vi "test_FirstSessionCloseErrors_CallCloseSessions_CloseCalledForAllSessions.vi"(8 "error in":errorcluster) -> (0 "error out":errorcluster, 2 "result":string, 3 "pass":bool)   [LabVIEW 2020, in "MeasurementServerTests.lvlib"]
uses:
  MeasurementServerTests.lvlib
  Runtime/Clients/Session Management V1/Session Reservation/Session Reservation.lvclass
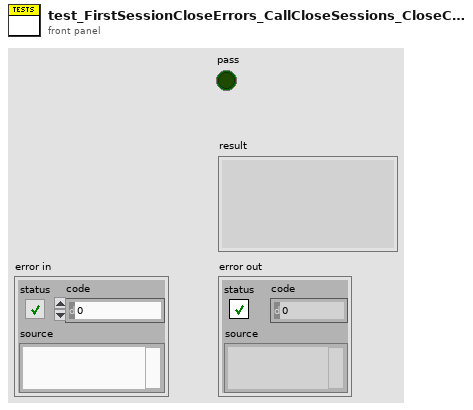
[diagram p1: front panel]
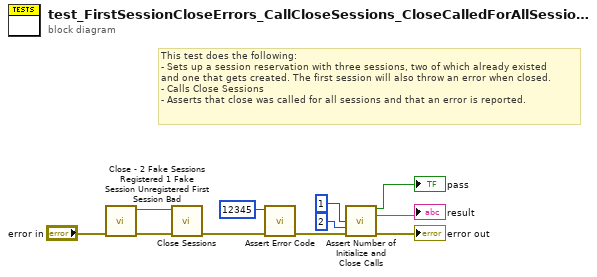
[diagram p0: block diagram]
diagram:
  # "This test does the following:\n- Sets up a session reservation with three sessions, two of which already existed\nand one that gets created. The first session will also throw an error when closed.\n- Calls Close Sessions\n- Asserts that close was called for all sessions and that an error is reported."
  n1 = call "Close - 2 Fake Sessions Registered 1 Fake Session Unregistered First Session Bad.vi"("error in"="error in") -> ("error out"=w10:errorcluster, "session reservation out"=w9:refnum<class "Session Reservation.lvclass">)  [unwired: 9 in]
  n2 = call "Close Sessions.vi"("error in"=w10, "session reservation in"=w9) -> ("error out"=w4:errorcluster)  [unwired: 8 in, 1 out]
  n3 = call "Assert Error Code.vi"("error in"=w4, "expected error code"=12345) -> ("error out"=w3:errorcluster)  [unwired: 7 in, 2 out]
  n4 = call "Assert Number of Initialize and Close Calls.vi"("expected close-close calls"=u32 1, "expected close-detach calls"=u32 2, "error in"=w3) -> ("pass"=→"pass":bool, "result"=→"result":string, "error out"=→"error out":errorcluster)  [unwired: 10 in]
